vi "PRO_Check Level.vi"(8 "Results In in":T2 {"Resistor" format="%.1f"; "Drain" format="%.3f"; "Fill" format="%.3f"}, 9 "Full Cfg":T3, 10 "Measurement":T1, 11 "ChA/!ChB":bool) -> (0 "Results In out":T2 {"Resistor" format="%.1f"; "Drain" format="%.3f"; "Fill" format="%.3f"})   [LabVIEW 2024]
uses:
  Control Definitions/Def Bench Status.ctl
  Control Definitions/Def PumpCtlRefs.ctl
  Control Definitions/Def BenchCfg.ctl
  Control Definitions/Def FullCfg.ctl
  Control Definitions/Def Results2.ctl
  Control Definitions/Def Xresult.ctl
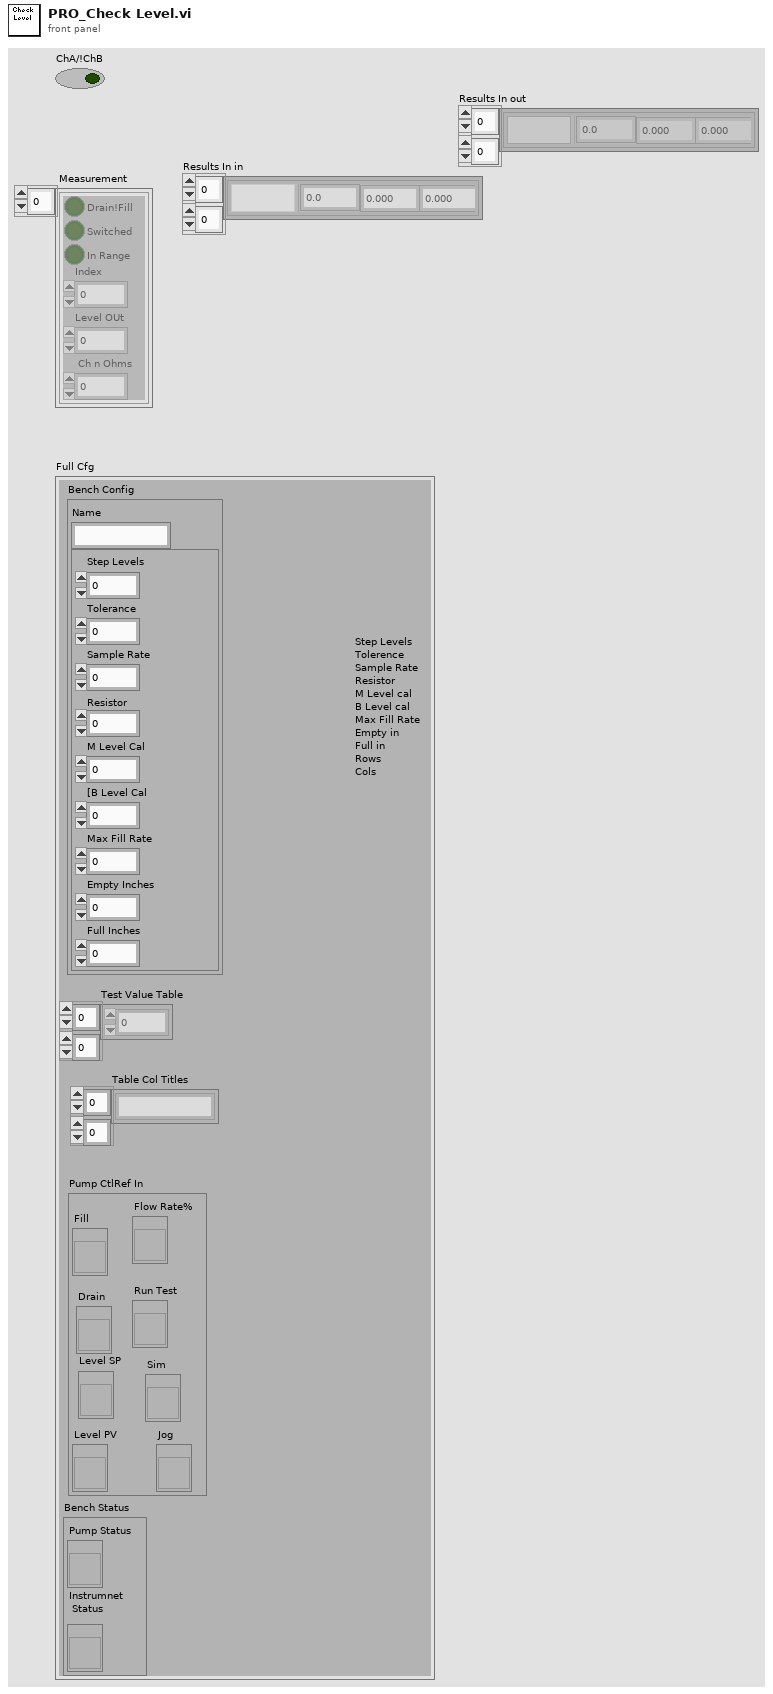
[diagram p1: front panel]
types:
  T1 = typedef "Def Xresult.ctl" = cluster{"Switched":bool, "In Range":bool, "Index":i16, "Level OUt":dbl, " Ch n Ohms":dbl, "Drain!Fill":bool}[]
  T2 = typedef "Def Results2.ctl" = cluster{"Fill":dbl, "Drain":dbl, "Status":i16, "Resistor":dbl}[][]
  T3 = typedef "Def FullCfg.ctl" = cluster{"Bench Config":T4, "Test Value Table ":dbl[][], "Table Col Titles":string[][], "Pump CtlRef In":T5, "Bench Status":T6}
  T4 = typedef "Def BenchCfg.ctl" = cluster{"Name":string, cluster{"Step Levels":dbl, "Tolerance":dbl, "Sample Rate":dbl, "Resistor":dbl, "M Level Cal":dbl, "[B Level Cal":dbl, "Max Fill Rate":dbl, "Empty Inches":dbl, "Full Inches":dbl}}
  T5 = typedef "Def PumpCtlRefs.ctl" = cluster{"Fill ":refnum<vi>, "Drain":refnum<vi>, "Level PV":refnum<vi>, "Flow Rate%":refnum<vi>, "Run Test":refnum<vi>, "Sim":refnum<vi>, "Jog":refnum<vi>, "Level SP":refnum<vi>}
  T6 = typedef "Def Bench Status.ctl" = cluster{"Pump Status":refnum<vi>, "Instrumnet\n Status":refnum<vi>}
  T7 = cluster{"Switched":bool, "In Range":bool, "Index":i16, "Level OUt":dbl, " Ch n Ohms":dbl, "Drain!Fill":bool}
  T8 = cluster{"Fill":dbl, "Drain":dbl, "Status":i16, "Resistor":dbl}
  T9 = typedef "Ded Spec RNG.ctl" = cluster{"Status":cluster{"ChA/!ChB":bool, "Drain/!Fill":bool, "In Range?":bool, "Switch Range?":bool, "Measure R?":bool}, "Specs":dbl[], "Indes":i32}
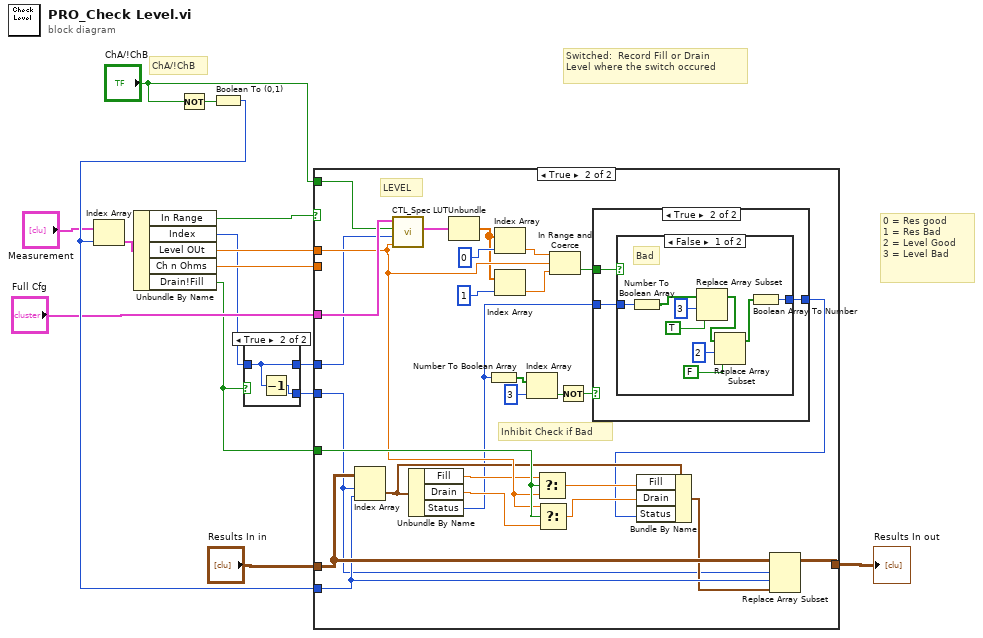
[diagram p0: block diagram]
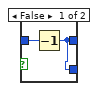
[diagram p2: hidden frame]
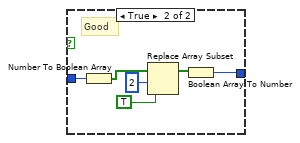
[diagram p5: hidden frame]
diagram:
  # "0 = Res good\n1 = Res Bad\n2 = Level Good\n3 = Level Bad"
  # "Switched:  Record Fill or Drain\nLevel where the switch occured"
  # "ChA/!ChB"
  n1 = Not(x="ChA/!ChB") -> (.not. x?=w15:bool)
  n2 = Boolean To (0,1)(Boolean=w15) -> (0, 1=w13:i16)
  n3 = Index Array(array="Measurement", index=w13) -> (element=w6:T7)
  n4 = Unbundle By Name(w6) -> ("In Range"=w11:bool, "Index"=w3:i16, "Level OUt"=w9:dbl, "Ch n Ohms"=w10:dbl, "Drain!Fill"=w4:bool)
  n5 = case shown="True" w4 {
    tunnel: w3 -> [w17 w19]
    tunnel: [w16 w19] -> w2
    tunnel: [w16 w18] -> w1
    frame False {
      n6 = Decrement(x=w17) -> (x-1=w16:i16)
    }
    frame True {
      n7 = Decrement(x=w19) -> (x-1=w18:i16)
    }
  }
  n8 = case shown="True" w11 {
    tunnel: "Full Cfg" -> [_ w44]
    tunnel: [w20 w48] -> w7
    tunnel: "Results In in" -> [w20 w47]
    tunnel: w9 -> [_ w39]
    tunnel: w10 -> [_ _]
    tunnel: w4 -> [_ w46]
    tunnel: w13 -> [_ w45]
    tunnel: "ChA/!ChB" -> [_ w31]
    tunnel: w2 -> [_ w23]
    tunnel: w1 -> [_ w22]
    frame False {
    }
    frame True {
      # "Inhibit Check if Bad"
      # "LEVEL"
      n9 = Index Array(array=w47, index (row)=w22, index (col)=w45) -> (element=w35:T8)
      n10 = call "CTL_Spec LUT.vi"("Level IN inches"=w39, "Index"=w23, "ChA/!ChB"=w31, "Full Cfg"=w44) -> ("Spec RNG"=w43:T9)  [unwired: 4 in, 3 out]
      n11 = Unbundle By Name(w35) -> ("Fill"=w37:dbl, "Drain"=w36:dbl, "Status"=w25:i16)
      n12 = Unbundle(w43) -> ("Specs"=w21:dbl[])  [unwired: 2 out]
      n13 = Number To Boolean Array(number=w25) -> (Boolean array=w28:bool[])
      n14 = Index Array(array=w21, index=0) -> (element=w40:dbl)
      n15 = Index Array(array=w21, index=1) -> (element=w41:dbl)
      n16 = Index Array(array=w28, index=3) -> (element=w26:bool)
      n17 = Select(t=w37, s=w46, f=w39) -> (s? t:f=w33:dbl)
      n18 = Select(t=w39, s=w46, f=w36) -> (s? t:f=w32:dbl)
      n19 = In Range and Coerce(upper limit=w40, x=w39, lower limit=w41) -> (In Range?=w30:bool)  [unwired: 1 out]
      n20 = Not(x=w26) -> (.not. x?=w24:bool)
      n21 = case shown="True" w24 {
        tunnel: w30 -> [_ w52]
        tunnel: [w49 w51] -> w29
        tunnel: w25 -> [w49 w50]
        frame False {
        }
        frame True {
          n22 = case shown="False" w52 {
            tunnel: w50 -> [w59 w65]
            tunnel: [w57 w62] -> w51
            frame False {
              # "Bad"
              n23 = Number To Boolean Array(number=w59) -> (Boolean array=w58:bool[])
              n24 = Replace Array Subset(array=w58, new element=TRUE ("new element/subarray"), index=3) -> (w54:bool[])
              n25 = Replace Array Subset(array=w54, new element=FALSE ("new element/subarray"), index=2) -> (w53:bool[])
              n26 = Boolean Array To Number(Boolean array=w53) -> (number=w57:u32)
            }
            frame True {
              # "Good"
              n27 = Number To Boolean Array(number=w65) -> (Boolean array=w64:bool[])
              n28 = Replace Array Subset(array=w64, new element=TRUE ("new element/subarray"), index=2) -> (w63:bool[])
              n29 = Boolean Array To Number(Boolean array=w63) -> (number=w62:u32)
            }
          }
        }
      }
      n30 = Bundle By Name(cluster=w35, "Fill"=w33, "Drain"=w32, "Status"=w29) -> (w34:T8)
      n31 = Replace Array Subset(array=w47, new element=w34, index (row)=w22, index (col)=w45) -> (w48:T2)
    }
  }
  "Results In out" <- w7
